vi "getSailingPoints.vi"(10 "sailing points left":i32, 11 "Waypoints":refnum<queue>) -> (2 "remaining sailing points?":bool, 3 "Array":refnum<class "Waypoint.lvclass">[](array[class]))   [LabVIEW 2013]
doc: "Extract remaining sailing points. If none left, returns an empty array."
uses:
  Classes/Waypoint/Waypoint.lvclass
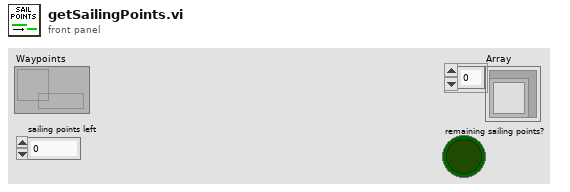
[diagram p1: front panel]
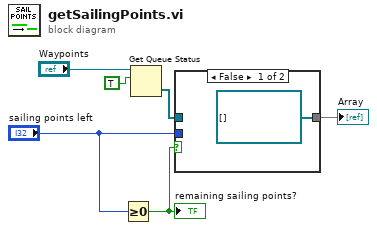
[diagram p0: block diagram]
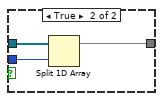
[diagram p2: hidden frame]
diagram:
  n1 = Greater Or Equal To 0?(x="sailing points left") -> (x >= 0?=w4:bool)
  "remaining sailing points?" <- w4
  n2 = Get Queue Status(queue="Waypoints", return elements? (F)=TRUE) -> (elements=w5:refnum<class "Waypoint.lvclass">[])  [unwired: 1 in, 7 out]
  n3 = case shown="False" w4 {
    tunnel: w5 -> [_ w10]
    tunnel: "sailing points left" -> [_ w9]
    tunnel: [refnum<class "Waypoint.lvclass">[] [] w8] -> w2
    frame False {
    }
    frame True {
      n4 = Split 1D Array(array=w10, index=w9) -> (first subarray=w8:refnum<class "Waypoint.lvclass">[])  [unwired: 1 out]
    }
  }
  "Array" <- w2
